vi "PWM Set Duty Cycle N Chans.vi"(8 "Error In":errorcluster, 9 "Duty Cycles":dbl[](array[numeric]), 10 "PWM Channels":u8[](array[numeric]), 11 "LINX Resource":T1) -> (0 "Error Out":errorcluster, 3 "LINX Resource":T1)   [LabVIEW 2014, in "LMH-LINX.lvlib"]
doc: "Set the duty cycle of the specified PWM channels. \n\nA duty cycle of 0 coresponds to 0% on and a duty cycle of 1 coresponds to 100% on."
uses:
  LMH-LINX.lvlib
  Private/Type Defs/LINX Ref.ctl
  Private/Type Defs/Platform.ctl
  Private/Type Defs/Interface.ctl
  Private/Device/Type Defs/LINX Device Config.ctl
  Private/Device/Type Defs/TCP Config.ctl
  Private/Device/Type Defs/Channels.ctl
  Private/Type Defs/Peripheral.ctl
  Private/Utilties/Generate Error.vi
  Private/Device/Device.lvlib
  Private/Local IO/Local IO.lvlib
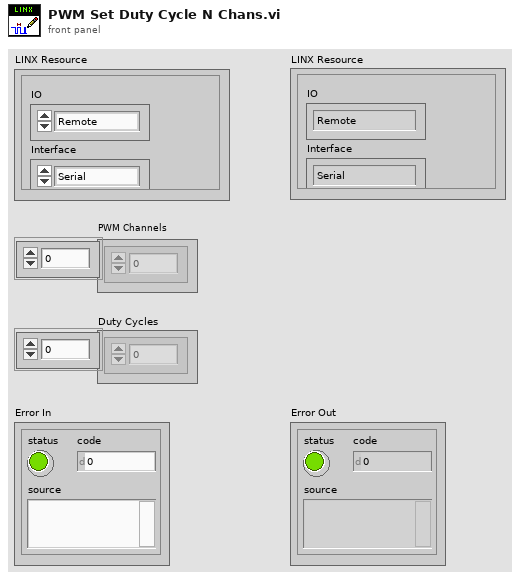
[diagram p1: front panel]
types:
  T1 = typedef "LMH-LINX.lvlib/LINX Ref.ctl" = cluster{"IO":T2, "Interface":T3, "LINX Device Config":T4}
  T2 = typedef "LMH-LINX.lvlib/Platform.ctl" = enum16{"Remote", "Local"}
  T3 = typedef "LMH-LINX.lvlib/Interface.ctl" = enum16{"Serial", "TCP"}
  T4 = typedef "LMH-LINX.lvlib/Device.lvlib/LINX Device Config.ctl" = cluster{"Interface":T3, "COM Port":refnum<visa-resource-name>, "TCP Configuration":T5, "Device Family":u8, "Device ID":u8, "Device Name":string, "TCP Ref":refnum<k5>, "Channels":T6}
  T5 = typedef "LMH-LINX.lvlib/Device.lvlib/TCP Config.ctl" = cluster{"IP Address":string, "Port":u16}
  T6 = typedef "LMH-LINX.lvlib/Channels.ctl" = cluster{"DI":u8[], "DO":u8[], "AI":u8[], "AO":u8[], "PWM":u8[], "QE":u8[], "UART":u8[], "I2C 2":u8[], "SPI":u8[], "CAN":u8[], "Servo":u8[], "AI Ref (V)":dbl, "AI Resolution (Bits)":u8, "AO Ref (V)":dbl, "AO Resolution (Bits)":u8}
  T7 = typedef "LMH-LINX.lvlib/Peripheral.ctl" = enum8{"DI", "DO", "AI", "AO", "PWM", "QE", "UART", "I2C", "SPI", "CAN", "Servo"}
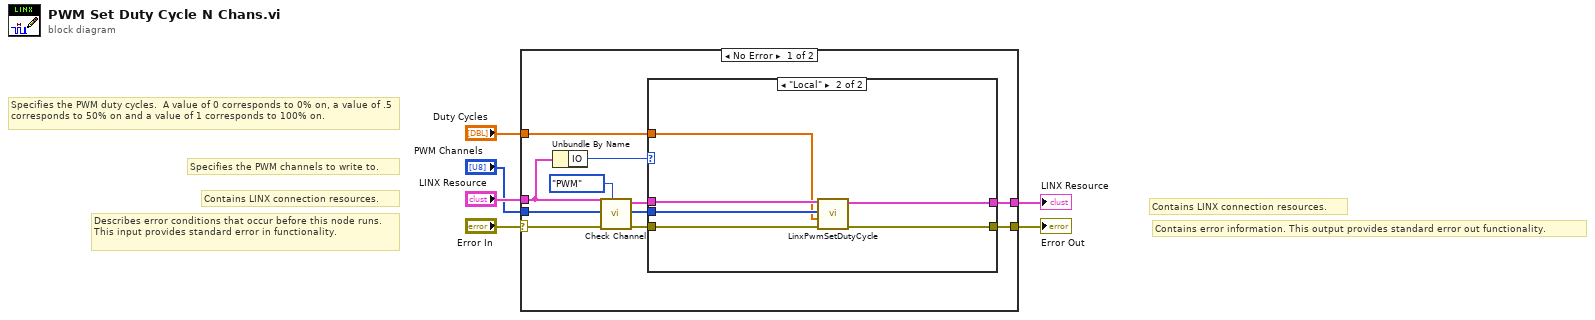
[diagram p0: block diagram]
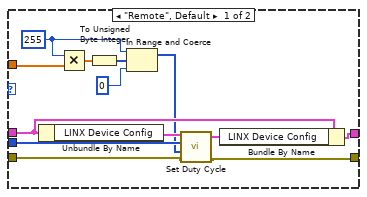
[diagram p2: hidden frame]
diagram:
  # "Specifies the PWM channels to write to."
  # "Specifies the PWM duty cycles.  A value of 0 corresponds to 0% on, a value of .5 corresponds to 50% on and a value of 1 corresponds to 100% on."
  # "Contains LINX connection resources."
  # "Contains error information. This output provides standard error out functionality."
  # "Contains LINX connection resources."
  # "Describes error conditions that occur before this node runs. This input provides standard error in functionality."
  n1 = case shown="No Error" "Error In" {
    selector: "Error In" -> [w7 w38]
    tunnel: [w16 w38] -> w6
    tunnel: [w15 w37] -> w5
    tunnel: "LINX Resource" -> [w13 w37]
    tunnel: "Duty Cycles" -> [w9 _]
    tunnel: "PWM Channels" -> [w8 _]
    frame No Error {
      n2 = Unbundle By Name(w13) -> ("IO"=w17:T2)
      n3 = call "Check Channel.vi"("Peripheral"=Peripheral."PWM", "Error In"=w7, "Channels"=w8, "LINX Resource"=w13) -> ("Error Out"=w11:errorcluster, "Channels"=w10:u8[], "LINX Resource"=w12:T1)  [unwired: 5 in]
      n4 = case shown="\"Local\"" w17 {
        tunnel: w11 -> [w27 w33]
        tunnel: w12 -> [w30 w34]
        tunnel: [w28 w36] -> w16
        tunnel: [w29 w35] -> w15
        tunnel: w9 -> [w19 w31]
        tunnel: w10 -> [w24 w32]
        frame "Remote", Default {
          w20 = u8 255
          n5 = Unbundle By Name(w30) -> ("LINX Device Config"=w25:T4)
          n6 = Multiply(x=w20, y=w19) -> (x*y=w23:dbl[])
          n7 = To Unsigned Byte Integer(number=w23) -> (unsigned 8bit integer=w22:u8[])
          n8 = In Range and Coerce(upper limit=w20, x=w22, lower limit=u8 0) -> (coerced(x)=w18:u8[])  [unwired: 1 out]
          n9 = call "Set Duty Cycle.vi"("Error In"=w27, "Duty Cycles (0-255)"=w18, "Channels"=w24, "LINX Device Config"=w25) -> ("Error Out"=w28:errorcluster, "LINX Device Config"=w26:T4)  [unwired: 6 in]
          n10 = Bundle By Name(cluster=w30, "LINX Device Config"=w26) -> (w29:T1)
        }
        frame "Local" {
          n11 = call "LinxPwmSetDutyCycle.vi"("Error In"=w33, "Duty Cycles"=w31, "PWM Channels"=w32, "LINX Resource"=w34) -> ("Error Out"=w36:errorcluster, "LINX Resource"=w35:T1)  [unwired: 6 in]
        }
      }
    }
    frame Error {
    }
  }
  "Error Out" <- w6
  "LINX Resource" <- w5
